vi "Email to Handler.vi"(8 "Email Handler IP":string, 9 "Message:":string, 10 "Subject:":string, 11 "To:":string) -> ()   [LabVIEW 2019]
panel:
  out "error out":errorcluster
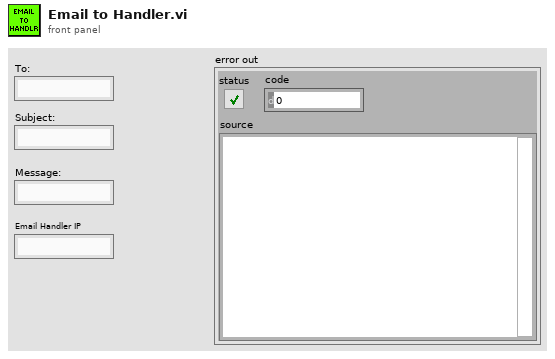
[diagram p1: front panel]
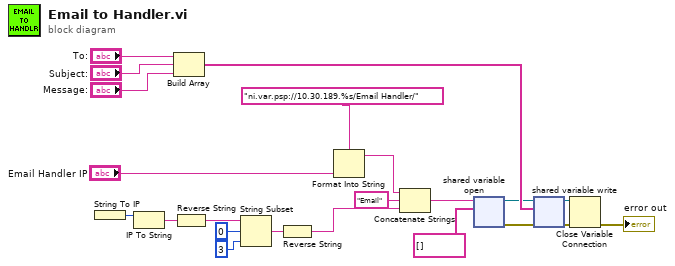
[diagram p0: block diagram]
diagram:
  n1 = String To IP() -> (0:w16:u32)  [unwired: 1 in]
  n2 = IP To String(2:w16) -> (0:w15:string)  [unwired: 1 in]
  n3 = Build Array("To:", "Subject:", "Message:") -> (w10:string[])
  n4 = Reverse String(1:w15) -> (0:w13:string)
  n5 = String Subset(string=w13, offset (0)=0, length (rest)=3 ("length (rest)")) -> (substring=w12:string)
  n6 = Reverse String(1:w12) -> (0:w11:string)
  n7 = Format Into String(format string="ni.var.psp://10.30.189.%s/Email Handler/", "Email Handler IP") -> (resulting string=w2:string)  [unwired: 2 in, 1 out]
  n8 = Concatenate Strings(w2, "Email" ("string"), w11) -> (w1:string)
  n9 = shared-variable-open(w1, string[] []) -> (w8:refnum<k21>, w6:errorcluster)  [unwired: 2 in]
  n10 = shared-variable-write(w8, w6, w10) -> (w9:refnum<k21>, w7:errorcluster)
  n11 = Close Variable Connection(8:w7, 11:w9) -> (0:→"error out":errorcluster)
